vi "PathToINIRequest.vi"(8 "error in (no error)":errorcluster, 11 "ModuleID":i32) -> (0 "error out":errorcluster)   [LabVIEW 2018, in "MyPluggableModule.lvlib"]
doc: "Sends a message from to return the path of the currently used confguration file."
uses:
  MyPluggableModule.lvlib
  PluginsShared/clEventType.ctl
  <vilib>/Utility/error.llb/Error Cluster From Error Code.vi
  <vilib>/ErrorRing/Error Ring.xnode
  PluginsShared/PluginsShared.lvlib
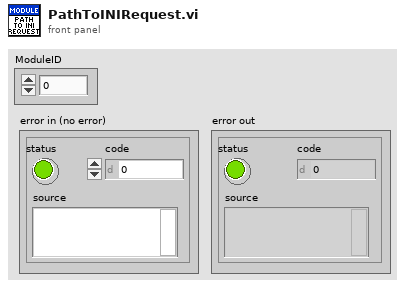
[diagram p1: front panel]
types:
  T1 = typedef "PluginsShared.lvlib/clRequestEvents.ctl" = cluster{"StopRequest":refnum<user-event>, "PathToINI":refnum<user-event>, " LoadPlugin":refnum<user-event>, "ShowPanel":refnum<user-event>, "PrefDlg":refnum<user-event>}
  T2 = typedef "PluginsShared.lvlib/clEventType.ctl" = cluster{"ModuleID":i32, "Data":variant}
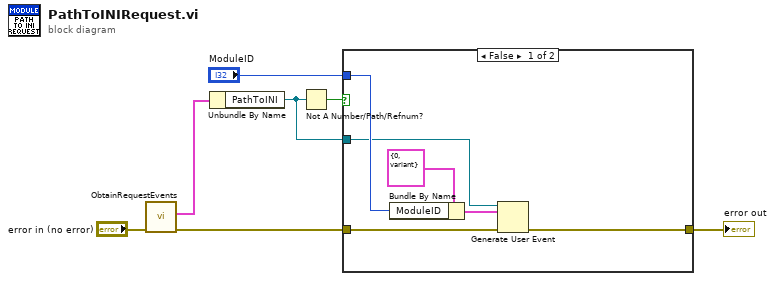
[diagram p0: block diagram]
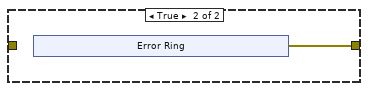
[diagram p2: hidden frame]
diagram:
  n1 = call "ObtainRequestEvents.vi"("error in (no error)"="error in (no error)") -> ("error out"=w1:errorcluster, "clRequestEvents"=w7:T1)  [unwired: 9 in]
  n2 = Unbundle By Name(w7) -> ("PathToINI"=w5:refnum<user-event>)
  n3 = Not A Number/Path/Refnum?(number/path/refnum=w5) -> (NaN/Path/Refnum?=w6:bool)
  n4 = case shown="False" w6 {
    tunnel: w5 -> [w10 _]
    tunnel: "ModuleID" -> [w12 _]
    tunnel: [w9 w14] -> w3
    tunnel: w1 -> [w8 _]
    frame False {
      n5 = Bundle By Name(cluster=T2 {"ModuleID"=0, "Data"=variant} ("clEventType"), "ModuleID"=w12) -> (w11:T2)
      n6 = Generate User Event(user event=w10, event data cluster=w11, error in=w8) -> (error out=w9:errorcluster)  [unwired: 1 in, 1 out]
    }
    frame True {
      n7 = xnode "Error Ring"() -> ("error out"=w14:errorcluster)
    }
  }
  "error out" <- w3
